vi "FB Core Mutate_1_1_1_0.vi"(8 "error in (no error)":errorcluster, 9 "Replies in":T16, 10 "Version":T18, 11 "Old State":T20) -> (0 "error out":errorcluster, 1 "Replies out":T16, 2 "Version Out":T18, 3 "New State":T20)   [LabVIEW 2020, in "FB Core.xnode"]
uses:
  <vilib>/functionblocks/FB Core/FB Core.xnode
  <vilib>/XNodeSupport/XNodeVariant.ctl
  <vilib>/XNodeSupport/XNodeVersion.ctl
  <vilib>/XNodeSupport/XNodeUShort.ctl
  <vilib>/XNodeSupport/XNodeStringArray.ctl
  <vilib>/XNodeSupport/XNodeString.ctl
  <vilib>/functionblocks/FB Core/FB Core State_old_1_0_0_0.ctl
  <vilib>/BlockNodeSupport/BlockNodeState.ctl
  <vilib>/BlockNodeSupport/TerminalData.ctl
  <vilib>/picture/picture.llb/imagedata.ctl
  <vilib>/functionblocks/FB Support/FB User State_old_1_0_0_0.ctl
  <vilib>/functionblocks/FB Support/FB Polymorphic Data.ctl
  <vilib>/functionblocks/FB Support/FB Terminal Data.ctl
  <vilib>/functionblocks/FB Support/FB Terminal Source.ctl
  <vilib>/functionblocks/FB Support/FB Variable Data.ctl
  <vilib>/functionblocks/FB Support/FB Variable Access.ctl
  <vilib>/functionblocks/FB Support/FB Terminal Wired State.ctl
  <vilib>/functionblocks/FB Support/FB Flavor.ctl
  <vilib>/functionblocks/FB Support/FB Error Conditions.ctl
  <vilib>/functionblocks/FB Core/FB Core State.ctl
  <vilib>/functionblocks/FB Support/FB User State.ctl
  <vilib>/XNodeSupport/NI_XNodeSupport.lvlib
panel:
  in  "State":T1 {"BlockNodeState"."Draw Style" items=["FunctionBlock", "ExpressVI", "Variable", "Elemental I/O", "32x32 Icon", "FunctionBlockCompact"]; "BlockNodeState"."Terminal Data"."Terminal Flags" format="%.0b"}
  in  "State_old_1_0_0_0":T14 {"BlockNodeState"."Draw Style" items=["FunctionBlock", "ExpressVI", "Variable", "Elemental I/O", "32x32 Icon", "FunctionBlockCompact"]; "BlockNodeState"."Terminal Data"."Terminal Flags" format="%.0b"}
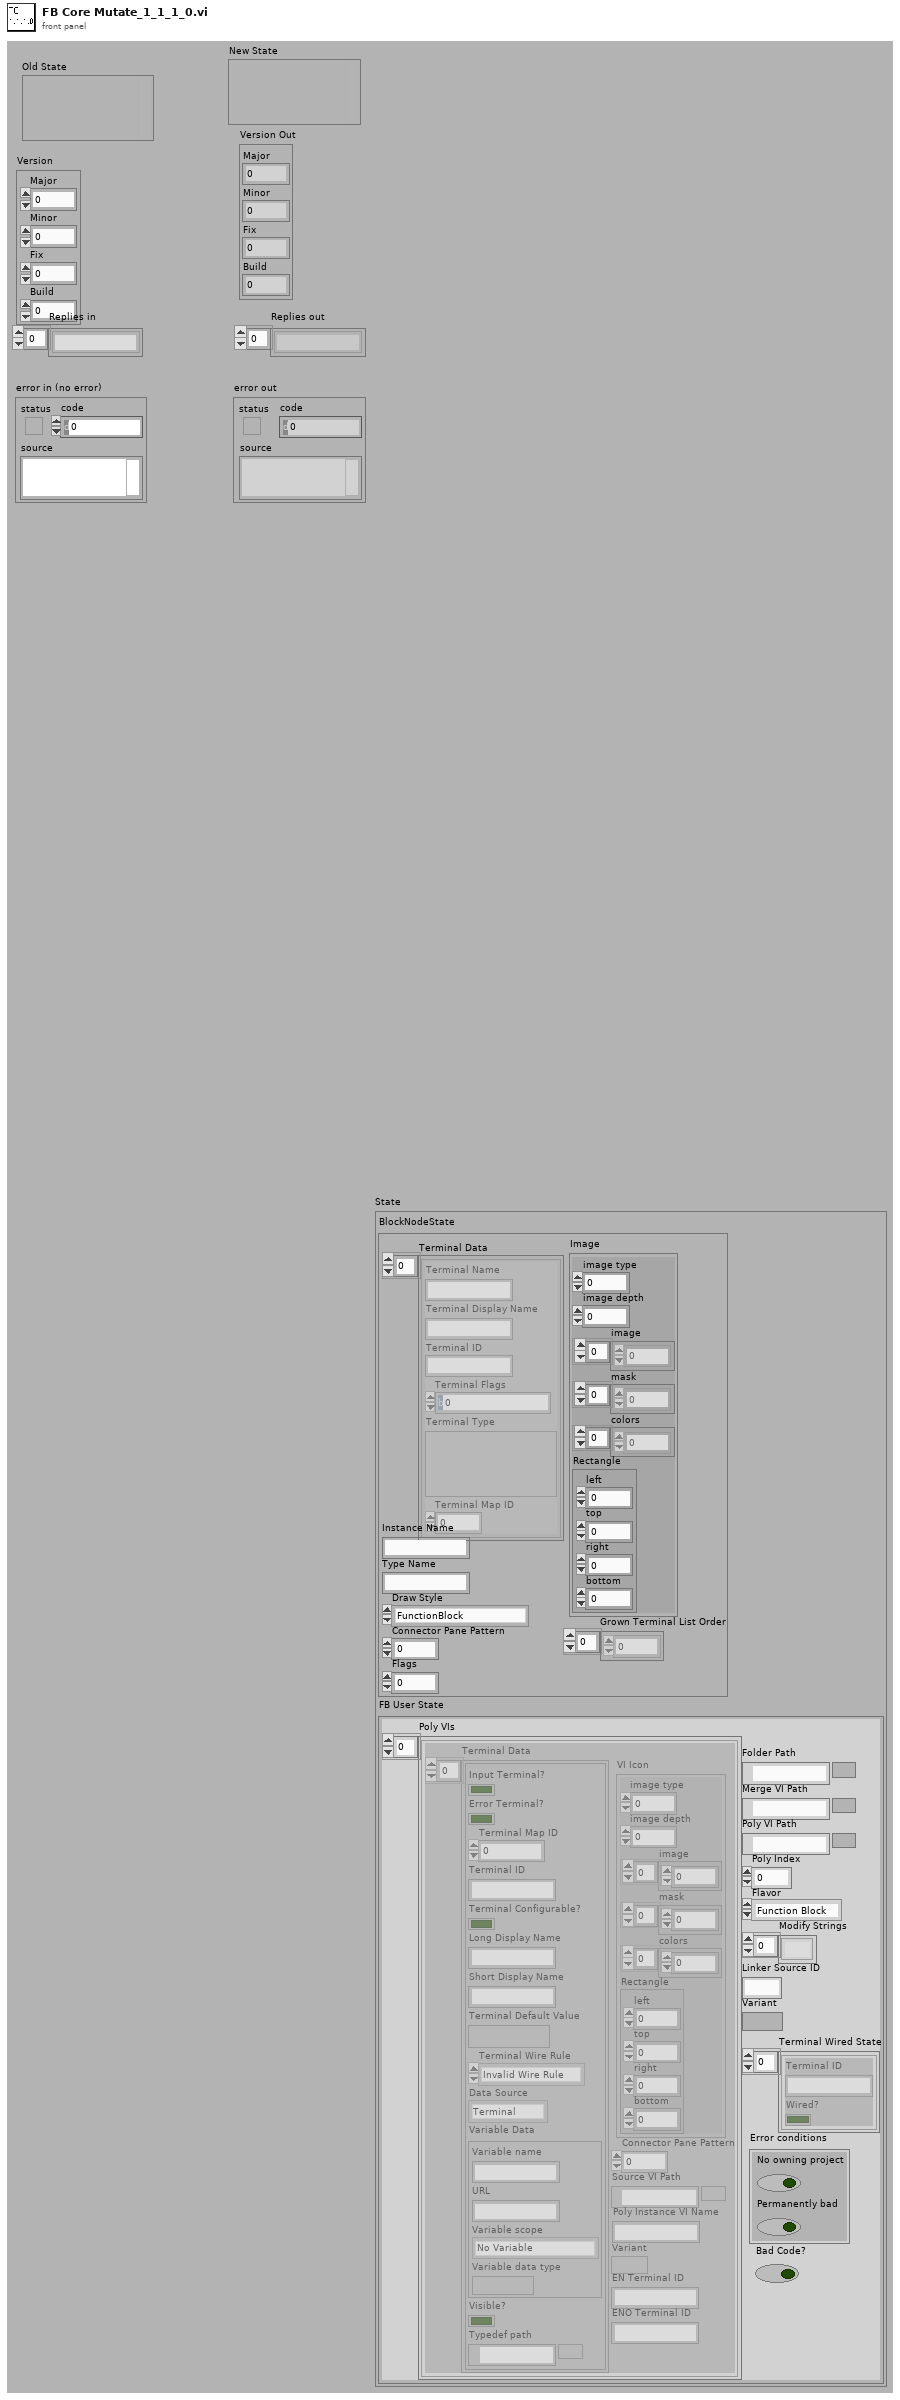
[diagram p1: front panel]
types:
  T1 = typedef "FB Core.xnode/FB Core State.ctl" = cluster{"BlockNodeState":T2, "FB User State":T5}
  T2 = typedef "BlockNodeState.ctl" = cluster{"Terminal Data":T3[], "Instance Name":string, "Type Name":string, "Draw Style":i32, "Connector Pane Pattern":i32, "Flags":i32, "Grown Terminal List Order":i32[], "Image":T4}
  T3 = typedef "TerminalData.ctl" = cluster{"Terminal Name":string, "Terminal Display Name":string, "Terminal ID":string, "Terminal Flags":i32, "Terminal Type":variant, "Terminal Map ID":i32}
  T4 = typedef "imagedata.ctl" = cluster{"image type":i32, "image depth":i32, "image":u8[], "mask":u8[], "colors":u32[], "Rectangle":cluster{"left":i16, "top":i16, "right":i16, "bottom":i16}}
  T5 = typedef "FB User State.ctl" = cluster{"Poly VIs":T6[], "Folder Path":path, "Merge VI Path":path, "Poly VI Path":path, "Linker Source ID":string, "Poly Index":i32, "Modify Strings":string[], "Terminal Wired State":T11[], "Variant":variant, "Flavor":T12, "Error conditions":T13, "Bad Code?":bool}
  T6 = typedef "FB Polymorphic Data.ctl" = cluster{"Terminal Data":T7[], "VI Icon":T4, "Connector Pane Pattern":u32, "Source VI Path":path, "Variant":variant, "EN Terminal ID":string, "ENO Terminal ID":string, "Poly Instance VI Name":string}
  T7 = typedef "FB Terminal Data.ctl" = cluster{"Input Terminal?":bool, "Error Terminal?":bool, "Terminal Map ID":i32, "Terminal ID":string, "Terminal Configurable?":bool, "Long Display Name":string, "Short Display Name":string, "Terminal Default Value":variant, "Terminal Wire Rule":enum16{"Invalid Wire Rule", "Required", "Recommended", "Optional", "Dynamic Dispatch"}, "Data Source":T8, "Variable Data":T9, "Visible?":bool, "Typedef path":path}
  T8 = typedef "FB Terminal Source.ctl" = enum16{"Terminal", "Variable", "Default"}
  T9 = typedef "FB Variable Data.ctl" = cluster{"Variable name":string, "URL":string, "Variable scope":T10, "Variable data type":variant}
  T10 = typedef "FB Variable Access.ctl" = enum16{"Unsupported", "No Variable", "Single-process", "Network-published"}
  T11 = typedef "FB Terminal Wired State.ctl" = cluster{"Terminal ID":string, "Wired?":bool}
  T12 = typedef "FB Flavor.ctl" = enum16{"Function Block", "Function"}
  T13 = typedef "FB Error Conditions.ctl" = cluster{"No owning project":bool, "Permanently bad":bool}
  T14 = typedef "FB Core.xnode/FB Core State_old_1_0_0_0.ctl" = cluster{"BlockNodeState":T2, "FB User State_old_1_0_0_0":T15}
  T15 = typedef "FB User State_old_1_0_0_0.ctl" = cluster{"Poly VIs":T6[], "Folder Path":path, "Merge VI Path":path, "Poly VI Path":path, "Linker Source ID":string, "Poly Index":i32, "Modify Strings":string[], "Terminal Wired State":T11[], "Variant":variant, "Flavor":T12, "Error conditions":T13}
  T16 = typedef "NI_XNodeSupport.lvlib/XNodeStringArray.ctl" = T17[]
  T17 = typedef "NI_XNodeSupport.lvlib/XNodeString.ctl" = string
  T18 = typedef "NI_XNodeSupport.lvlib/XNodeVersion.ctl" = cluster{"Major":T19, "Minor":T19, "Fix":T19, "Build":T19}
  T19 = typedef "NI_XNodeSupport.lvlib/XNodeUShort.ctl" = u16
  T20 = typedef "NI_XNodeSupport.lvlib/XNodeVariant.ctl" = variant
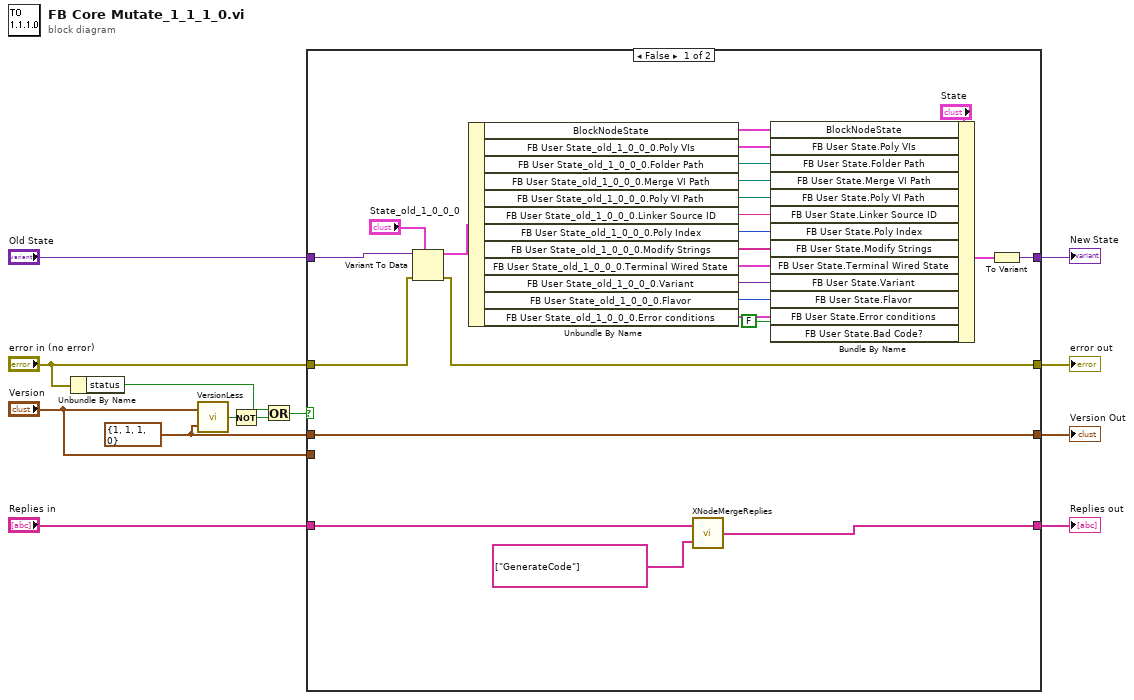
[diagram p0: block diagram]
diagram:
  w12 = T18 {"Major"=1, "Minor"=1, "Fix"=1, "Build"=0} ("y")
  n1 = Unbundle By Name("error in (no error)") -> ("status"=w4:bool)
  n2 = call <vilib>:"VersionLess.vi"("y"=w12, "x"="Version") -> ("x < y?"=w13:bool)
  n3 = Not(x=w13) -> (.not. x?=w3:bool)
  n4 = Or(x=w4, y=w3) -> (x .or. y?=w6:bool)
  n5 = case shown="False" w6 {
    tunnel: w12 -> [w38 _]
    tunnel: [w36 w42] -> w11
    tunnel: "Old State" -> [w37 w42]
    tunnel: [w38 w41] -> w9
    tunnel: "Version" -> [_ w41]
    tunnel: [w33 w40] -> w7
    tunnel: "error in (no error)" -> [w34 w40]
    tunnel: [w30 w39] -> w2
    tunnel: "Replies in" -> [w31 w39]
    frame False {
      n6 = Variant To Data(error in=w34, type="State_old_1_0_0_0", Variant=w37) -> (data=w32:T14, error out=w33:errorcluster)
      n7 = Unbundle By Name(w32) -> ("BlockNodeState"=w28:T2, "FB User State_old_1_0_0_0.Poly VIs"=w26:T6[], "FB User State_old_1_0_0_0.Folder Path"=w25:path, "FB User State_old_1_0_0_0.Merge VI Path"=w24:path, "FB User State_old_1_0_0_0.Poly VI Path"=w23:path, "FB User State_old_1_0_0_0.Linker Source ID"=w22:string, "FB User State_old_1_0_0_0.Poly Index"=w21:i32, "FB User State_old_1_0_0_0.Modify Strings"=w20:string[], "FB User State_old_1_0_0_0.Terminal Wired State"=w19:T11[], "FB User State_old_1_0_0_0.Variant"=w18:variant, "FB User State_old_1_0_0_0.Flavor"=w17:T12, "FB User State_old_1_0_0_0.Error conditions"=w16:T13)
      n8 = call <vilib>:"XNodeMergeReplies.vi"("New Replies"=string[] ["GenerateCode"], "Old Replies"=w31) -> ("Merged Replies"=w30:string[])
      n9 = Bundle By Name(cluster="State", "BlockNodeState"=w28, "FB User State.Poly VIs"=w26, "FB User State.Folder Path"=w25, "FB User State.Merge VI Path"=w24, "FB User State.Poly VI Path"=w23, "FB User State.Linker Source ID"=w22, "FB User State.Poly Index"=w21, "FB User State.Modify Strings"=w20, "FB User State.Terminal Wired State"=w19, "FB User State.Variant"=w18, "FB User State.Flavor"=w17, "FB User State.Error conditions"=w16, "FB User State.Bad Code?"=FALSE) -> (w35:T1)
      n10 = To Variant(anything=w35) -> (Variant=w36:variant)
    }
    frame True {
      # "Either there was an error in,\nor the version is not less than 1.0.0.6.\nPass input values out."
    }
  }
  "New State" <- w11
  "Version Out" <- w9
  "error out" <- w7
  "Replies out" <- w2
